vi "resize camera space image to SLM space.vi"(5 "Y SLM":i32=1080, 7 "X SLM":i32=1080, 8 "error in (no error)":errorcluster, 9 "Y camera":i32=625, 10 "X camera":i32=1035, 11 "original image":T1) -> (0 "error out":errorcluster, 3 "Resized image":T1)   [LabVIEW 2025]
uses:
  <vilib>/vision/Image Controls.llb/IMAQ Image.ctl
  <vilib>/vision/NI_Vision_Development_Module.lvlib
panel:
  out "Image 2":T1(plugin-control)
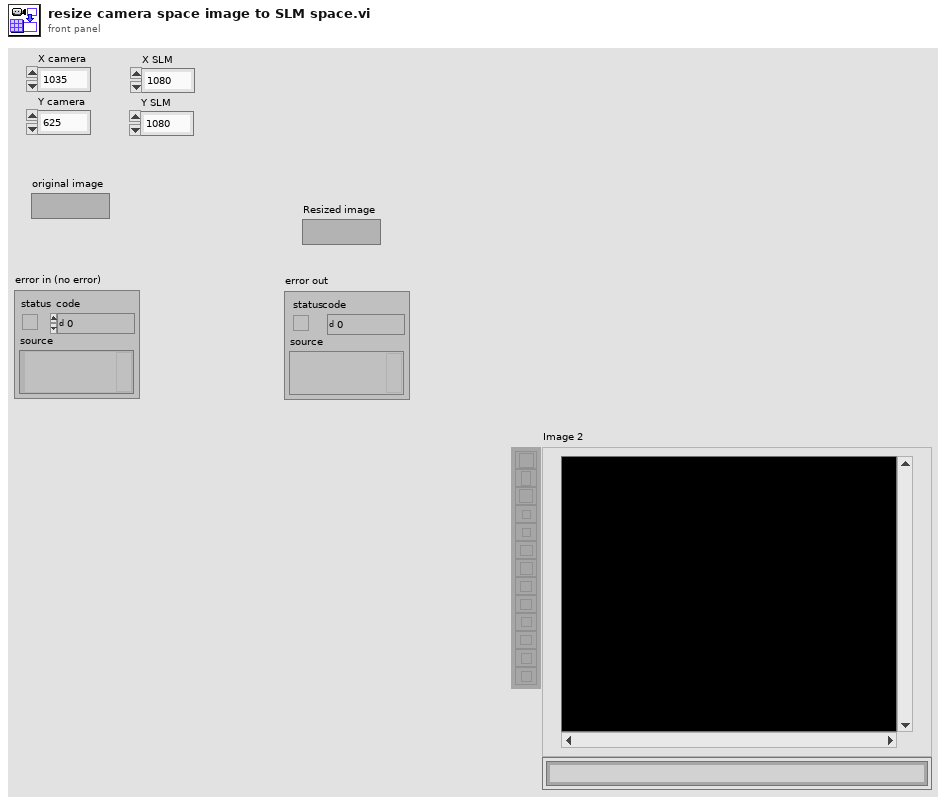
[diagram p1: front panel]
types:
  T1 = typedef "IMAQ Image.ctl" = refnum<image>
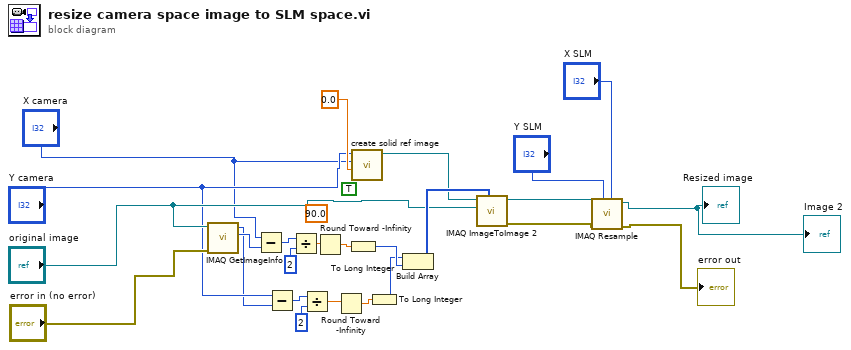
[diagram p0: block diagram]
diagram:
  (unwired) 90.0 ("Angle (degrees)")
  (unwired) TRUE ("Maintain Size")
  n1 = call "IMAQ GetImageInfo"("error in (no error)"="error in (no error)", "Image"="original image") -> ("Y Resolution"=w2:i32, "X Resolution"=w1:i32)  [unwired: 2 in, 6 out]
  n2 = Subtract(x="X camera", y=w2) -> (x-y=w25:i32)
  n3 = Subtract(x="Y camera", y=w1) -> (x-y=w22:i32)
  n4 = Divide(x=w25, y=2) -> (x/y=w23:dbl)
  n5 = Divide(x=w22, y=2) -> (x/y=w20:dbl)
  n6 = Round Toward -Infinity(1:w23) -> (0:w19:dbl)
  n7 = Round Toward -Infinity(1:w20) -> (0:w18:dbl)
  n8 = To Long Integer(number=w19) -> (32bit integer=w4:i32)
  n9 = call "create solid ref image.vi"("Pixel Value (default 255)"=sgl 0.0, "Y resolution"="X camera", "X resolution"="Y camera") -> ("solid image"=w7:T1)  [unwired: 7 in, 1 out]
  n10 = To Long Integer(number=w18) -> (32bit integer=w3:i32)
  n11 = Build Array(w3, w4) -> (w15:i32[])
  n12 = call "IMAQ ImageToImage 2"("Offset Left/Top"=w15, "Image Src (Small)"="original image", "Image Src (Large)"=w7) -> ("error out"=w9:errorcluster, "Image Dst Out"=w8:T1)  [unwired: 7 in]
  n13 = call "IMAQ Resample"("X Resolution"="X SLM", "Y Resolution"="Y SLM", "error in (no error)"=w9, "Image Src"=w8) -> ("error out"=→"error out":errorcluster, "Image Dst Out"=→"Resized image" →"Image 2":T1)  [unwired: 6 in]
